vi "PLC_to_Auto.vi"() -> ()   [LabVIEW 2017]
panel:
  out "Recipe selected":bool
  out "ST1 COUNTER NG RESET":bool
  out "ST1 COUNTER OK RESET":bool
  out "ST1 data save":bool
  out "ST1 scn rslt":bool
  in  "UPDATE THREAD LOCKER DELAY":bool
  out "AUTO SCREEN":bool
  out "MANUAL":bool
  out "PLC Communication STATION 1":bool
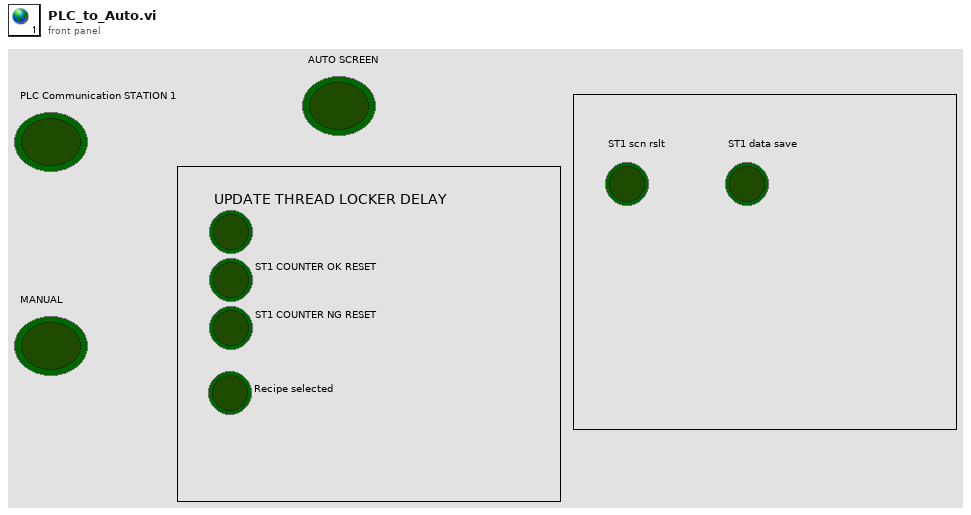
[diagram p1: front panel]
diagram:
